vi "CNV Vector Builder.vi"(11 "Cluster":cluster{"WiBCI16T Data out":T1, "En MAP":u16} {"WiBCI16T Data out"."Reg Map"."ADS2" format="%x"; "WiBCI16T Data out"."Reg Map"."ADS1" format="%x"}) -> ()   [LabVIEW 2016, in "CML UI.lvlib"]
uses:
  CML UI.lvlib
  Acquisition/WiBCI16T_Data.ctl
  Acquisition/WiBCI16T_Status.ctl
  Acquisition/Reg_Map.ctl
  Acquisition/Acquisition.lvlib
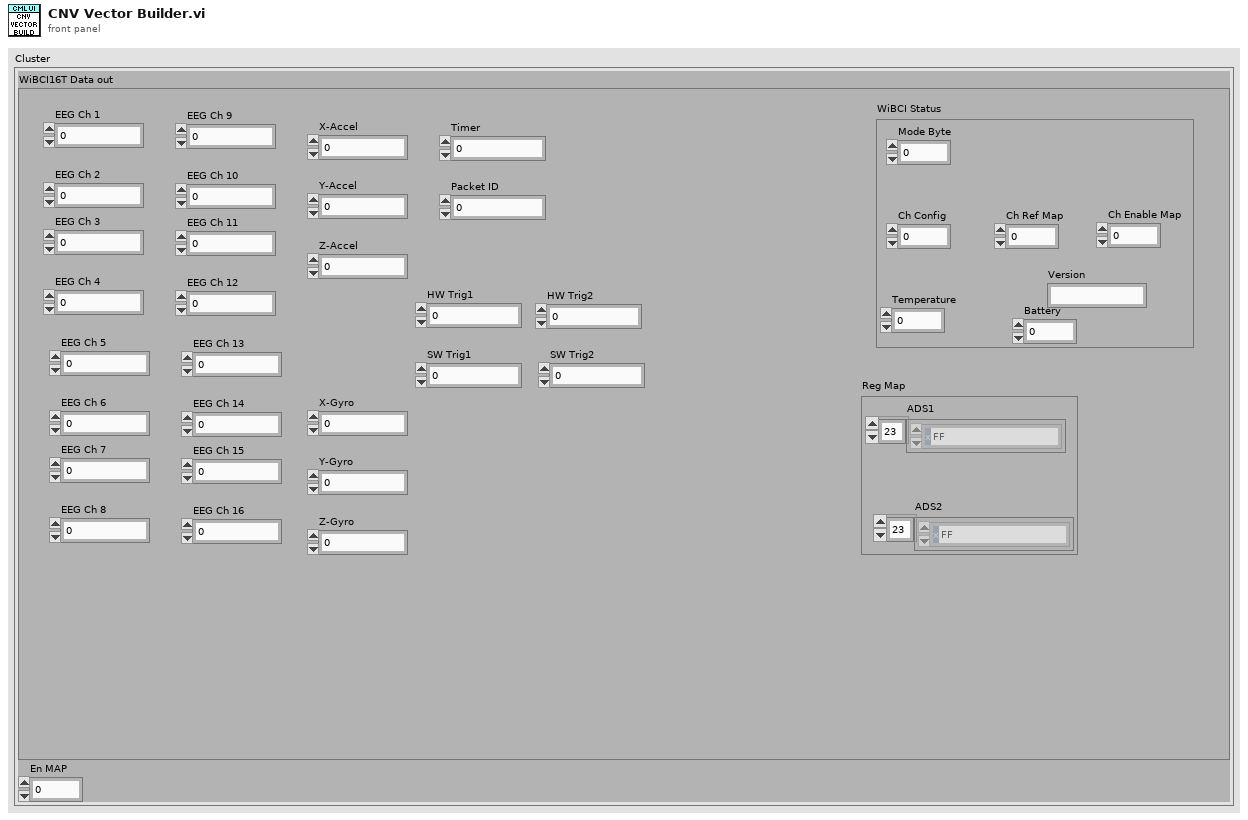
[diagram p1: front panel]
types:
  T1 = typedef "Acquisition.lvlib/WiBCI16T_Data.ctl" = cluster{"EEG Ch 1":dbl, "EEG Ch 2":dbl, "EEG Ch 3":dbl, "EEG Ch 4":dbl, "EEG Ch 5":dbl, "EEG Ch 6":dbl, "EEG Ch 7":dbl, "EEG Ch 8":dbl, "EEG Ch 9":dbl, "EEG Ch 10":dbl, "EEG Ch 11":dbl, "EEG Ch 12":dbl, "EEG Ch 13":dbl, "EEG Ch 14":dbl, "EEG Ch 15":dbl, "EEG Ch 16":dbl, "X-Accel":i16, "Y-Accel":i16, "Z-Accel":i16, "X-Gyro":i16, "Y-Gyro":i16, "Z-Gyro":i16, "Timer":u32, "Packet ID":u32, "HW Trig1":u8, "SW Trig1":i8, "HW Trig2":u8, "SW Trig2":i8, "WiBCI Status":T2, "Reg Map":T3}
  T2 = typedef "Acquisition.lvlib/WiBCI16T_Status.ctl" = cluster{"Mode Byte":u8, "Ch Config":u8, "Ch Ref Map":u16, "Ch Enable Map":u16, "Temperature":sgl, "Battery":u8, "Version":string}
  T3 = typedef "Acquisition.lvlib/Reg_Map.ctl" = cluster{"ADS1":u8[], "ADS2":u8[]}
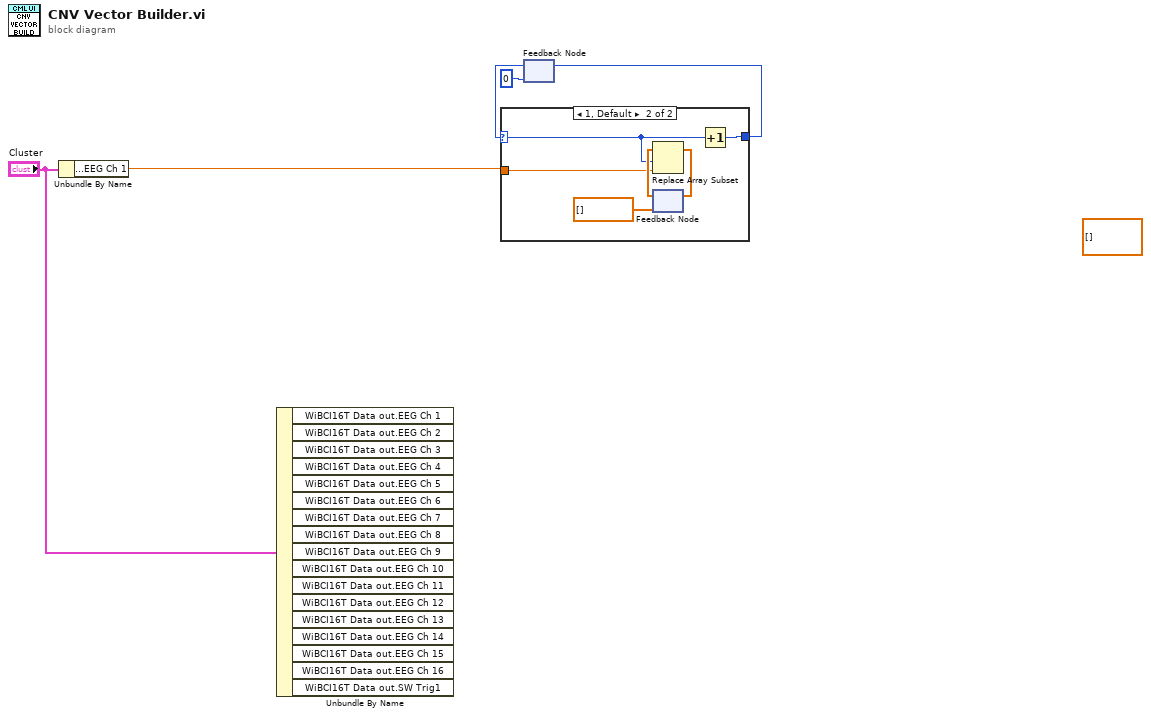
[diagram p0: block diagram]
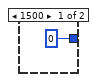
[diagram p2: hidden frame]
diagram:
  (unwired) dbl[][] [] ("appended array")
  n1 = Unbundle By Name("Cluster") -> ("WiBCI16T Data out.EEG Ch 1"=w5:dbl)
  n2 = Unbundle By Name("Cluster") -> ()  [unwired: 17 out]
  n3 = feedback #1(u16 0) -> (w3:u16)
  n4 = case shown="1, Default" w3 {
    selector: w3 -> [_ w8]
    tunnel: w5 -> [_ w10]
    tunnel: [u16 0 w9] -> w4
    frame 1500 {
    }
    frame 1, Default {
      n5 = feedback #2(dbl[] [] ("appended array")) -> (w11:dbl[])
      n6 = Replace Array Subset(array=w11, new element=w10, index=w8) -> (w7:dbl[])
      n7 = feedback-in #2(w7) -> ()
      n8 = Increment(x=w8) -> (x+1=w9:u16)
    }
  }
  n9 = feedback-in #1(w4) -> ()
